vi "7_wfm_graph.vi"() -> ()   [LabVIEW 2017]
panel:
  out "Waveform Graph 4":dbl[][](graph)
  out "Waveform Graph 3":dbl[](graph)
  out "Waveform Graph 2":cluster{i32, dbl, dbl[]}(graph)
  out "Waveform Graph 1":dbl[](graph)
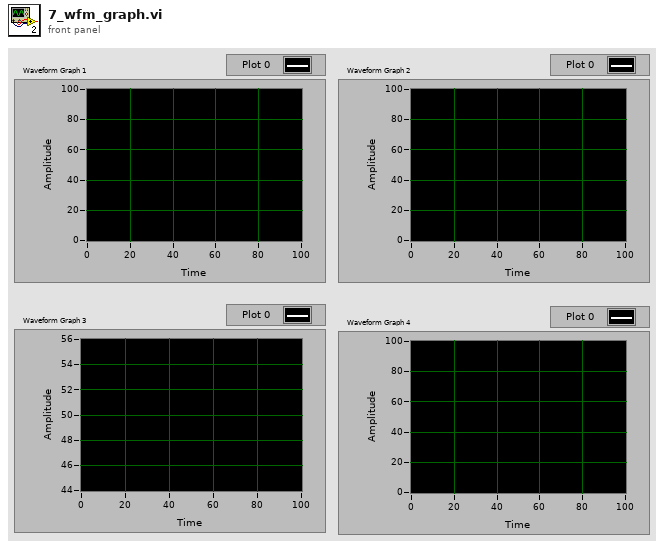
[diagram p1: front panel]
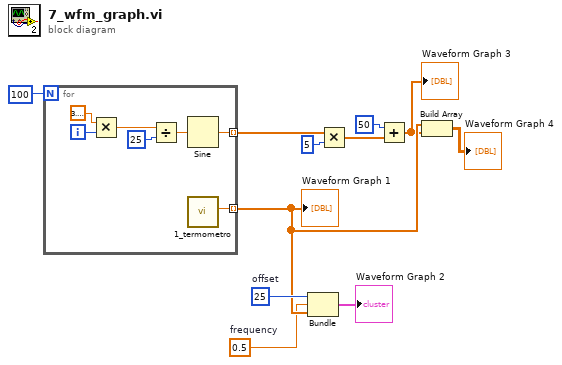
[diagram p0: block diagram]
diagram:
  w1 = 0.5  # frequency
  w9 = 25  # offset
  n1 = for {
    N: 100 -> [_]
    tunnel: [w18] -> w7 mode=indexing
    tunnel: [w12] -> w6 mode=indexing
    i -> [w16]
    n2 = Multiply(x=3.141592653589793, y=w16) -> (x*y=w17:dbl)
    n3 = Divide(x=w17, y=25) -> (x/y=w13:dbl)
    n4 = Sine(x=w13) -> (sin(x)=w12:dbl)
    n5 = call "1_termometro.vi"() -> ("Celsius"=w18:dbl)  [unwired: 1 in, 3 out]
  }
  "Waveform Graph 1" <- w7
  n6 = Bundle("offset"=w9, "frequency"=w1, w7) -> (→"Waveform Graph 2":cluster{"offset":i32, "frequency":dbl, dbl[]})  [unwired: 1 in]
  n7 = Multiply(x=w6, y=5) -> (x*y=w5:dbl[])
  n8 = Add(x=50, y=w5) -> (x+y=w3:dbl[])
  "Waveform Graph 3" <- w3
  n9 = Build Array(w7, w3) -> (→"Waveform Graph 4":dbl[][])
